vi "cycle.vi"() -> ()   [LabVIEW 2018]
uses:
  <vilib>/DAQmx/create/channels.llb/DAQmx Create Channel (AI-Voltage-Basic).vi
  <vilib>/DAQmx/configure/timing.llb/DAQmx Timing (Sample Clock).vi
  <resource>/objmgr/daqmx.rc
panel:
  in  "samples per channel":i32=1000
  in  "sample mode":i32(ring)=10178 items=["Finite Samples"=10178, "Continuous Samples"=10123, "Hardware Timed Single Point"=12522]
  in  "rate":dbl=1000.0 format="%0.2f"
  in  "scale name":tag
  in  "scale name":tag
  in  "scale name":tag
  in  "scale name":tag
  in  "channels 4":tag
  in  "channels 3":tag
  in  "channels 2":tag
  in  "channels 1":tag
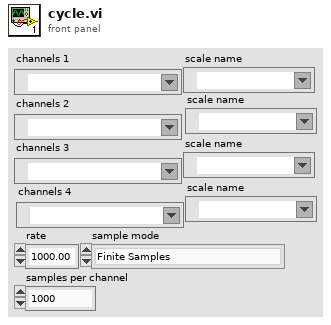
[diagram p1: front panel]
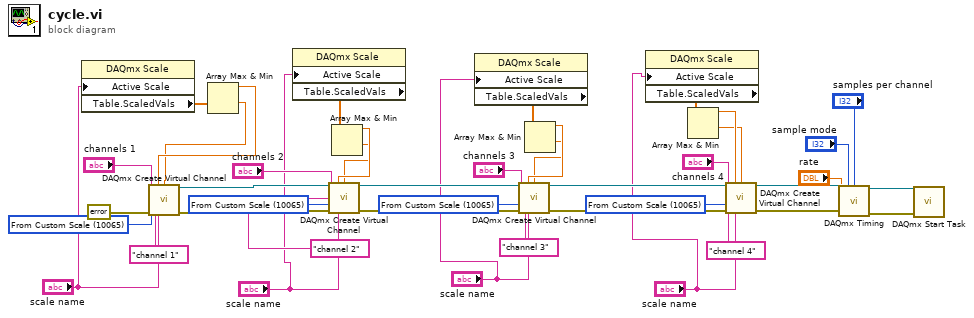
[diagram p0: block diagram]
diagram:
  w8 = 10065 items=["Volts"=10348, "From Custom Scale"=10065] ("units")
  w9 = 10065 items=["Volts"=10348, "From Custom Scale"=10065] ("units")
  w10 = 10065 items=["Volts"=10348, "From Custom Scale"=10065] ("units")
  w11 = 10065 items=["Volts"=10348, "From Custom Scale"=10065] ("units")
  n1 = property class="DAQmx Scale"("Active Scale"="scale name") -> ("Table.ScaledVals"=w27:dbl[])  [unwired: 2 in, 2 out]
  n2 = Array Max & Min(array=w27) -> (max value=w25:dbl, min value=w24:dbl)  [unwired: 2 out]
  n3 = call-poly <vilib>:"DAQmx Create Virtual Channel.vi"("maximum value"=w25, "minimum value"=w24, "physical channels"="channels 1", "name to assign"="channel 1", "units"=w11, "error in"=errorcluster {"status"=FALSE, "code"=0, "source"=""}, "custom scale name"="scale name") -> ("task out"=w34:refnum<k21>, "error out"=w29:errorcluster)  [unwired: 7 in]
  n4 = property class="DAQmx Scale"("Active Scale"="scale name") -> ("Table.ScaledVals"=w23:dbl[])  [unwired: 2 in, 2 out]
  n5 = Array Max & Min(array=w23) -> (max value=w19:dbl, min value=w18:dbl)  [unwired: 2 out]
  n6 = call-poly <vilib>:"DAQmx Create Virtual Channel.vi"("task in"=w34, "maximum value"=w19, "minimum value"=w18, "physical channels"="channels 2", "name to assign"="channel 2", "units"=w10, "error in"=w29, "custom scale name"="scale name") -> ("task out"=w33:refnum<k21>, "error out"=w30:errorcluster)  [unwired: 6 in]
  n7 = property class="DAQmx Scale"("Active Scale"="scale name") -> ("Table.ScaledVals"=w22:dbl[])  [unwired: 2 in, 2 out]
  n8 = Array Max & Min(array=w22) -> (max value=w16:dbl, min value=w15:dbl)  [unwired: 2 out]
  n9 = call-poly <vilib>:"DAQmx Create Virtual Channel.vi"("task in"=w33, "maximum value"=w16, "minimum value"=w15, "physical channels"="channels 3", "name to assign"="channel 3", "units"=w9, "error in"=w30, "custom scale name"="scale name") -> ("task out"=w32:refnum<k21>, "error out"=w31:errorcluster)  [unwired: 6 in]
  n10 = property class="DAQmx Scale"("Active Scale"="scale name") -> ("Table.ScaledVals"=w21:dbl[])  [unwired: 2 in, 2 out]
  n11 = Array Max & Min(array=w21) -> (max value=w13:dbl, min value=w12:dbl)  [unwired: 2 out]
  n12 = call-poly <vilib>:"DAQmx Create Virtual Channel.vi"("task in"=w32, "maximum value"=w13, "minimum value"=w12, "physical channels"="channels 4", "name to assign"="channel 4", "units"=w8, "error in"=w31, "custom scale name"="scale name") -> ("task out"=w7:refnum<k21>, "error out"=w6:errorcluster)  [unwired: 6 in]
  n13 = call-poly <vilib>:"DAQmx Timing.vi"("task/channels in"=w7, "sample mode"="sample mode", "samples per channel"="samples per channel", "rate"="rate", "error in"=w6) -> ("task out"=w2:refnum<k21>, "error out"=w1:errorcluster)  [unwired: 9 in]
  n14 = call <vilib>:"DAQmx Start Task.vi"("task/channels in"=w2, "error in"=w1) -> ()  [unwired: 12 in, 2 out]
